vi "server stop notifier.vi"(2 "notifier in":refnum<notifier>, 3 "action":enum16{"get", "set"}(ring)=enum."set") -> (0 "notifier out":refnum<notifier>)   [LabVIEW 2016, in "JSONRPC Server.lvclass"]
uses:
  JSONRPC Server.lvclass
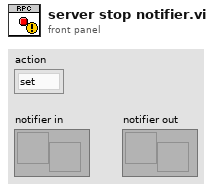
[diagram p1: front panel]
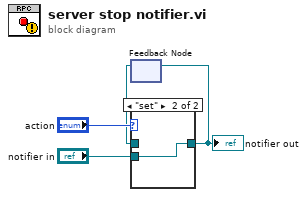
[diagram p0: block diagram]
diagram:
  n1 = feedback #1() -> (w2:refnum<notifier>)  [unwired: 1 in]
  n2 = case shown="\"set\"" "action" {
    tunnel: w2 -> [w5 _]
    tunnel: [w5 w6] -> w3
    tunnel: "notifier in" -> [_ w6]
    frame "get", Default {
    }
    frame "set" {
    }
  }
  "notifier out" <- w3
  n3 = feedback-in #1(w3) -> ()
